vi "code.vi"(11 "字符串输入":string) -> (3 "字符串输出":string)   [LabVIEW 2016, in "Alarm interface.lvlib"]
uses:
  Alarm interface.lvlib
panel:
  in  "关闭":bool
  in  "确定":bool
  out "上限":u32
  out "下限":u32
  # "code"
  # "~"
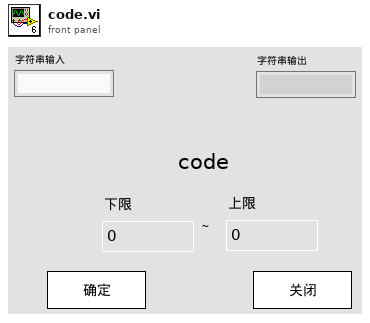
[diagram p1: front panel]
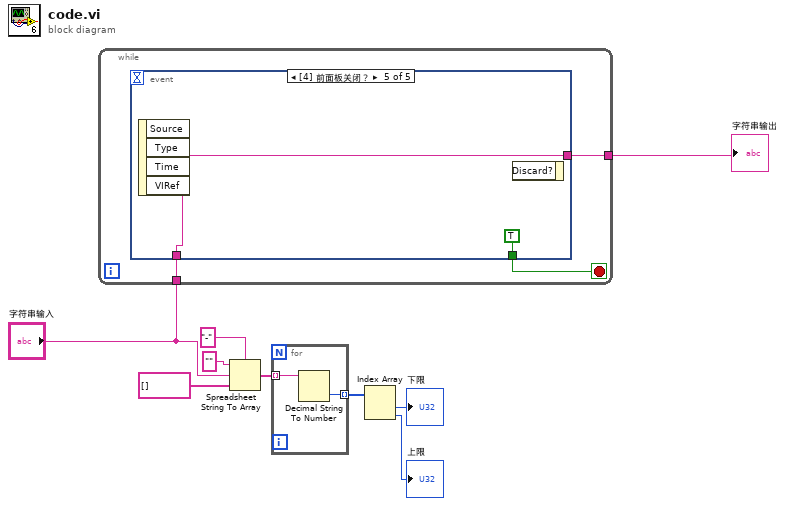
[diagram p0: block diagram]
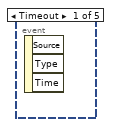
[diagram p2: hidden frame]
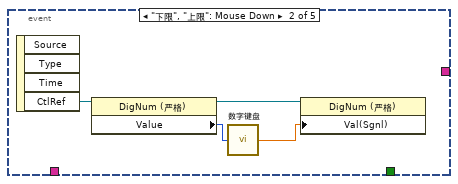
[diagram p3: hidden frame]
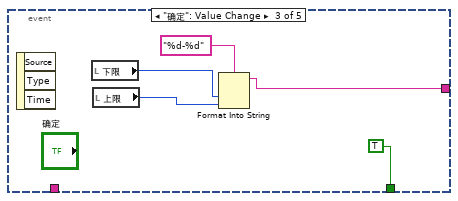
[diagram p4: hidden frame]
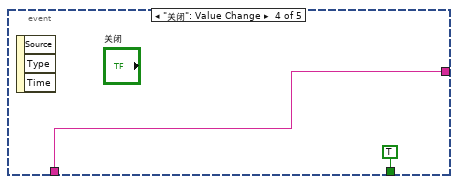
[diagram p5: hidden frame]
diagram:
  n1 = while {
    tunnel: [w11] -> w2
    tunnel: "字符串输入" -> [w10]
    stop <- w12 stop-if-true
    n2 = event shown="[4] 前面板关闭？" {
      selector: _ -> [_ _ _ _ _]
      dyn-events: _ -> [_ _ _ _ _]
      timeout: _ -> [_ _ _ _ _]
      tunnel: [_ _ TRUE TRUE TRUE] -> w12
      tunnel: [_ _ w17 w22 w24] -> w11
      tunnel: w10 -> [_ _ _ w22 w24]
      event Timeout {
        n3 = event-data() -> ()  [unwired: 1 in, 3 out]
      }
      event "下限", "上限": Mouse Down {
        n4 = event-data() -> ("CtlRef"=w16:refnum<vi>)  [unwired: 1 in, 3 out]
        n5 = property class="DigNum (严格)"(reference=w16) -> (reference out=w14:refnum<vi>, "Value"=w15:u32)  [unwired: 1 in, 1 out]
        n6 = call "数字键盘.vi"("OldNumber"=w15) -> ("NewNumber"=w13:sgl)
        n7 = property class="DigNum (严格)"(reference=w14, "Val(Sgnl)"=w13) -> ()  [unwired: 1 in, 2 out]
      }
      event "确定": Value Change {
        n8 = event-data() -> ()  [unwired: 1 in, 3 out]
        n9 = local read "下限"() -> (w20:u32)
        n10 = local read "上限"() -> (w19:u32)
        n11 = Format Into String(format string="%d-%d" ("格式字符串"), w20, w19) -> (resulting string=w17:string)  [unwired: 2 in, 1 out]
      }
      event "关闭": Value Change {
        n12 = event-data() -> ()  [unwired: 1 in, 3 out]
      }
      event Panel Close? {
        n13 = event-data() -> ()  [unwired: 1 in, 4 out]
        n14 = event-data() -> ()  [unwired: 2 in, 1 out]
      }
    }
  }
  "字符串输出" <- w2
  n15 = Spreadsheet String To Array(delimiter (Tab)="-" ("分隔符(Tab)"), format string="" ("格式字符串"), spreadsheet string="字符串输入", array type (2D Dbl)=string[] []) -> (array=w6:string[])
  n16 = for {
    tunnel: w6 -> [w27] mode=indexing
    tunnel: [w26] -> w5 mode=indexing
    n17 = Decimal String To Number(string=w27) -> (number=w26:i32)  [unwired: 2 in, 1 out]
  }
  n18 = Index Array(array=w5) -> (element #1=→"下限":i32, element #2=→"上限":i32)  [unwired: 2 in]
